vi "Color SensorVI.vi"() -> (1 "Normalized Color":cluster{"R":dbl, "G":dbl, "B":dbl}, 2 "Color":u32(colorbox))   [LabVIEW 2019]
uses:
  <vilib>/Rock Robotics/SystemInterfaces/i2clib/i2c_bus.ctl
panel:
  out "color":dbl
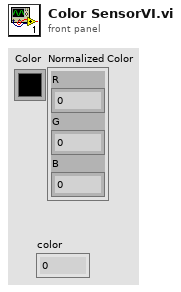
[diagram p1: front panel]
types:
  T1 = typedef "i2c_bus.ctl" = enum16{"I2C On-Board", "I2C MXP", "Invalid"}
  T2 = typedef "Color Sensor V3 DevRef.ctl" = cluster{"I2CDevRef":T3}
  T3 = typedef "WPI_I2CDevRef.ctl" = cluster{"DevStatus":errorcluster, "Device Address":u8, "Handle":i32, "I2C Bus":T1}
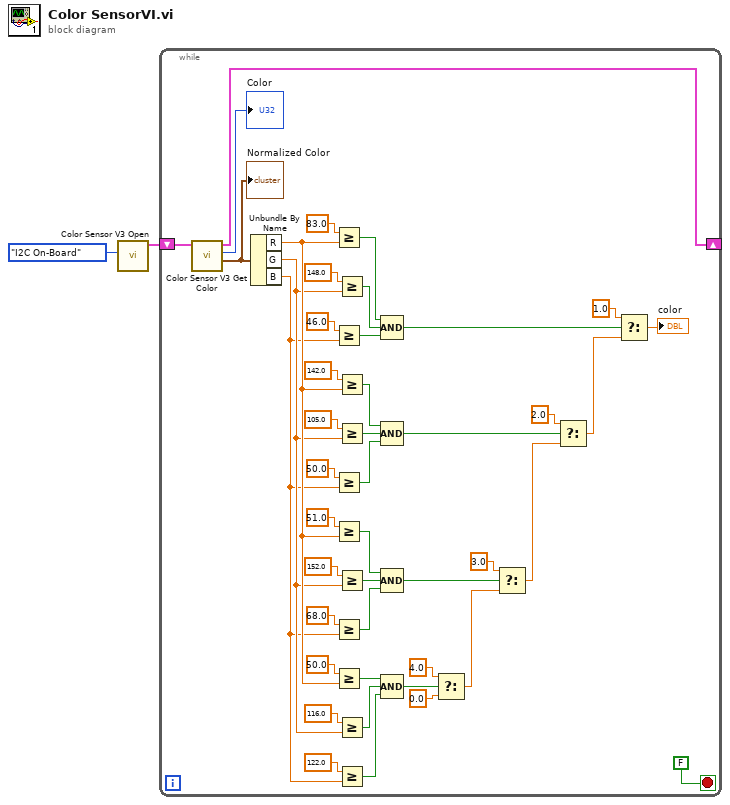
[diagram p0: block diagram]
diagram:
  n1 = call <vilib>:"Color Sensor V3 Open.vi"("I2C Bus"=i2c_bus."I2C On-Board") -> ("ColorSensorDevRef"=w1:T2)  [unwired: 9 in, 1 out]
  n2 = while {
    shift-right: [w46] -> _
    shift-left: w1 -> [w47]
    stop <- FALSE stop-if-true
    n3 = call <vilib>:"Color Sensor V3 Get Color.vi"("ColorSensorDevRef"=w47) -> ("Normalized Color"=w43:cluster{"R":dbl, "G":dbl, "B":dbl}, "Color"=→"Color":u32, "ColorSensorDevRef out"=w46:T2)  [unwired: 7 in, 1 out]
    "Normalized Color" <- w43
    n4 = Unbundle By Name(w43) -> ("R"=w12:dbl, "G"=w11:dbl, "B"=w10:dbl)
    n5 = Greater Or Equal?(x=83.0 ("R"), y=w12) -> (x >= y?=w32:bool)
    n6 = Greater Or Equal?(x=46.0 ("B"), y=w10) -> (x >= y?=w34:bool)
    n7 = Greater Or Equal?(x=50.0 ("B"), y=w10) -> (x >= y?=w24:bool)
    n8 = Greater Or Equal?(x=51.0 ("R"), y=w12) -> (x >= y?=w17:bool)
    n9 = Greater Or Equal?(x=68.0 ("B"), y=w10) -> (x >= y?=w19:bool)
    n10 = Greater Or Equal?(x=50.0 ("R"), y=w12) -> (x >= y?=w7:bool)
    n11 = Greater Or Equal?(x=148.0 ("G"), y=w11) -> (x >= y?=w33:bool)
    n12 = Greater Or Equal?(x=142.0 ("R"), y=w12) -> (x >= y?=w26:bool)
    n13 = Greater Or Equal?(x=105.0 ("G"), y=w11) -> (x >= y?=w25:bool)
    n14 = Greater Or Equal?(x=152.0 ("G"), y=w11) -> (x >= y?=w18:bool)
    n15 = Greater Or Equal?(x=116.0 ("G"), y=w11) -> (x >= y?=w8:bool)
    n16 = Greater Or Equal?(x=122.0 ("B"), y=w10) -> (x >= y?=w9:bool)
    n17 = Compound Arithmetic op=AND(w32, w33, w34) -> (w31:bool)
    n18 = Compound Arithmetic op=AND(w26, w25, w24) -> (w23:bool)
    n19 = Compound Arithmetic op=AND(w17, w18, w19) -> (w16:bool)
    n20 = Compound Arithmetic op=AND(w7, w8, w9) -> (w6:bool)
    n21 = Select(t=4.0, s=w6, f=0.0) -> (s? t:f=w41:dbl)
    n22 = Select(t=3.0, s=w16, f=w41) -> (s? t:f=w40:dbl)
    n23 = Select(t=2.0, s=w23, f=w40) -> (s? t:f=w39:dbl)
    n24 = Select(t=1.0, s=w31, f=w39) -> (s? t:f=→"color":dbl)
  }
